vi "Move.vi"(8 "error in (no error)":errorcluster, 9 "Absolute (T)":bool=TRUE, 10 "Point":refnum<class "Point.lvclass">, 11 "Triangle in":refnum<class "Triangle.lvclass">) -> (0 "error out":errorcluster, 3 "Triangle out":refnum<class "Triangle.lvclass">)   [LabVIEW 2021, in "Picture2D.lvlib" / "Triangle.lvclass"]
uses:
  Triangle.lvclass
  Polygone/Polygone.lvclass
  Shape/Shape.lvclass
  Point/Point.lvclass
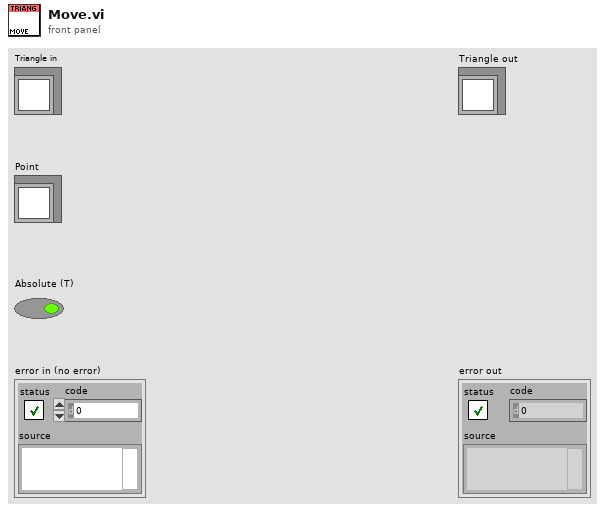
[diagram p1: front panel]
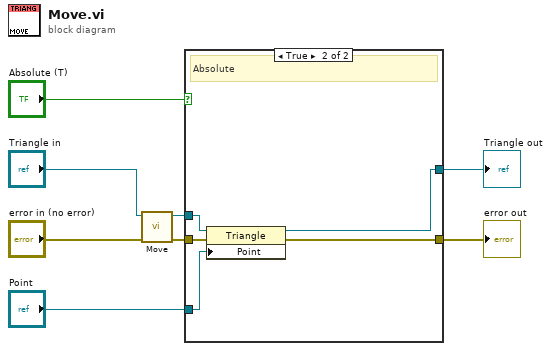
[diagram p0: block diagram]
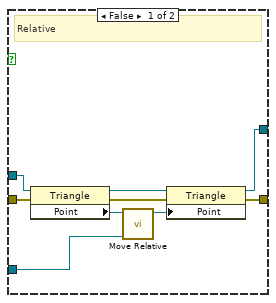
[diagram p2: hidden frame]
diagram:
  n1 = call-parent "Move.vi"("error in (no error)"="error in (no error)", "Shape in"="Triangle in") -> ("error out"=w8:errorcluster, "Shape out"=w7:refnum<class "Triangle.lvclass">)  [unwired: 8 in]
  n2 = case shown="True" "Absolute (T)" {
    tunnel: w7 -> [w17 w22]
    tunnel: [w13 w21] -> w5
    tunnel: w8 -> [w12 w20]
    tunnel: [w10 w19] -> w4
    tunnel: "Point" -> [w9 w18]
    frame False {
      # "Relative"
      n3 = property class="Triangle"(reference=w17, error in=w12) -> (reference out=w14:refnum<class "Triangle.lvclass">, error out=w11:errorcluster, "Point"=w16:refnum<class "Point.lvclass">)
      n4 = call "Move Relative.vi"("Move"=w9, "Point"=w16) -> ("New Point"=w15:refnum<class "Point.lvclass">)  [unwired: 9 in]
      n5 = property class="Triangle"(reference=w14, error in=w11, "Point"=w15) -> (reference out=w13:refnum<class "Triangle.lvclass">, error out=w10:errorcluster)
    }
    frame True {
      # "Absolute"
      n6 = property class="Triangle"(reference=w22, error in=w20, "Point"=w18) -> (reference out=w21:refnum<class "Triangle.lvclass">, error out=w19:errorcluster)
    }
  }
  "error out" <- w4
  "Triangle out" <- w5
